vi "Smooth.vi"(10 "Window Size":i32=3, 11 "X":dbl[](array[numeric])) -> (3 "subarray":dbl[](array[numeric]))   [LabVIEW 2011]
uses:
  <vilib>/Analysis/4window.llb/Flat Top Window (DBL).vi
  <vilib>/Analysis/2dsp.llb/1D Convolution (DBL).vi
  <vilib>/Analysis/NI_AALPro.lvlib
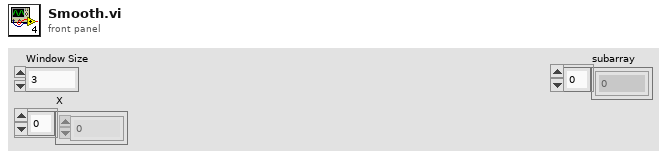
[diagram p1: front panel]
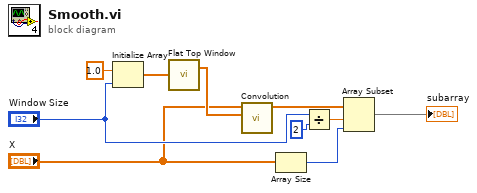
[diagram p0: block diagram]
diagram:
  n1 = Initialize Array(1.0 ("element"), "Window Size") -> (w10:dbl[])
  n2 = call-poly <vilib>:"Flat Top Window.vi"("X"=w10) -> ("Windowed X"=w8:dbl[])  [unwired: 1 out]
  n3 = call-poly <vilib>:"Convolution.vi"("Y"=w8, "X"="X") -> ("X * Y"=w2:dbl[])  [unwired: 8 in, 1 out]
  n4 = Array Size(array="X") -> (size(s)=w4:i32)
  n5 = Divide(x="Window Size", y=2) -> (x/y=w7:dbl)
  n6 = Array Subset(array=w2, index=w7, length=w4) -> (→"subarray":dbl[])
